vi "PQconnect.vi"(7 "encoding":string, 8 "conninfo":string) -> (0 "PQprotocolVersion":u32, 1 "PQerrorMessage":string, 2 "PQStatus":T1(ring)=enum."CONNECTION_BAD", 3 "conn":u32)   [LabVIEW 2017, in "libpqutility.lvlib"]
doc: "Establish PostgreSQL database connection. See PostgreSQL c-lib dokumentation for further information."
uses:
  libpqutility.lvlib
  libpqlv/libpqlv.lvlib
panel:
  out "PQsetClientEncoding":i32
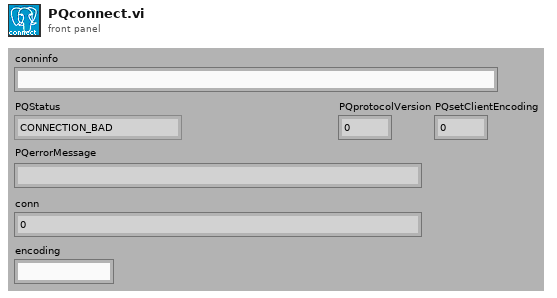
[diagram p1: front panel]
types:
  T1 = enum16{"CONNECTION_OK", "CONNECTION_BAD", "CONNECTION_STARTED", "CONNECTION_MADE", "CONNECTION_AWAITING_RESPONSE", "CONNECTION_AUTH_OK", "CONNECTION_SETENV", "CONNECTION_SSL_STARTUP", "CONNECTION_NEEDED"}
  T2 = enum32{"CONNECTION_OK", "CONNECTION_BAD", "CONNECTION_STARTED", "CONNECTION_MADE", "CONNECTION_AWAITING_RESPONSE", "CONNECTION_AUTH_OK", "CONNECTION_SETENV", "CONNECTION_SSL_STARTUP", "CONNECTION_NEEDED"}
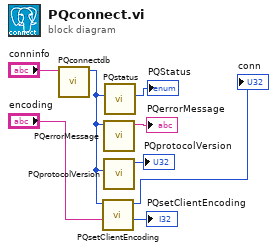
[diagram p0: block diagram]
diagram:
  n1 = call "PQconnectdb.vi"("conninfo"="conninfo") -> ("conn"=w3:u32)  [unwired: 9 in, 1 out]
  n2 = call "PQsetClientEncoding.vi"("encode"="encoding", "conn"=w3) -> ("PQsetClientEncoding"=→"PQsetClientEncoding":i32, "conn_out"=→"conn":u32)  [unwired: 8 in]
  n3 = call "PQerrorMessage.vi"("conn"=w3) -> ("PQerrorMessage"=→"PQerrorMessage":string)  [unwired: 8 in, 2 out]
  n4 = call "PQprotocolVersion.vi"("conn"=w3) -> ("PQprotocolVersion"=→"PQprotocolVersion":u32)  [unwired: 9 in, 1 out]
  n5 = call "PQstatus.vi"("conn"=w3) -> ("PQStatus"=→"PQStatus":T2)  [unwired: 9 in, 1 out]
